vi "获取操作日志 (子VI).vi"(11 "table输入":string(combo)) -> ()   [LabVIEW 2016, in "数据传输系统.lvlib"]
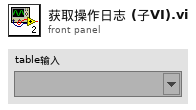
[diagram p1: front panel]
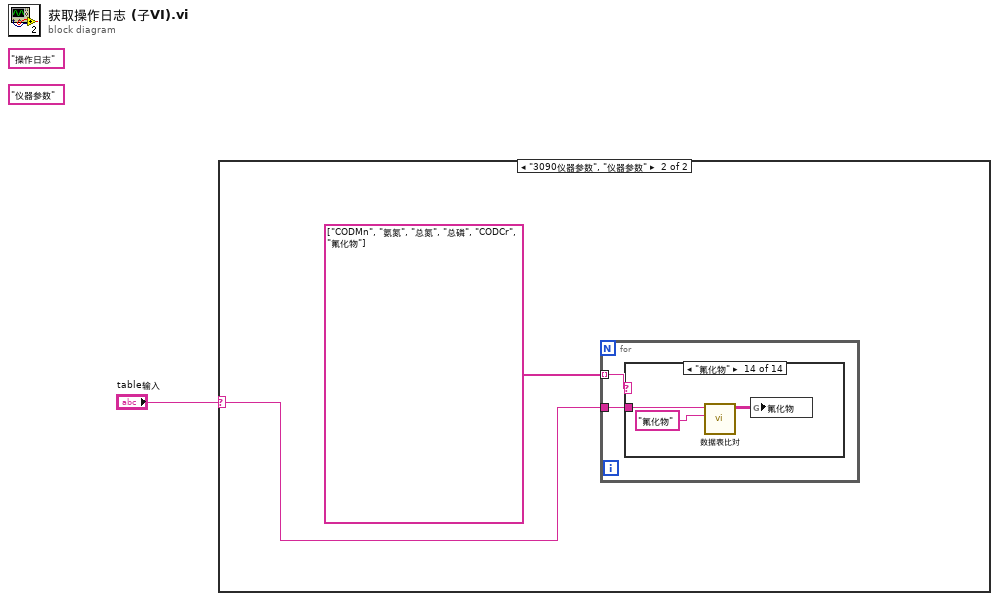
[diagram p0: block diagram]
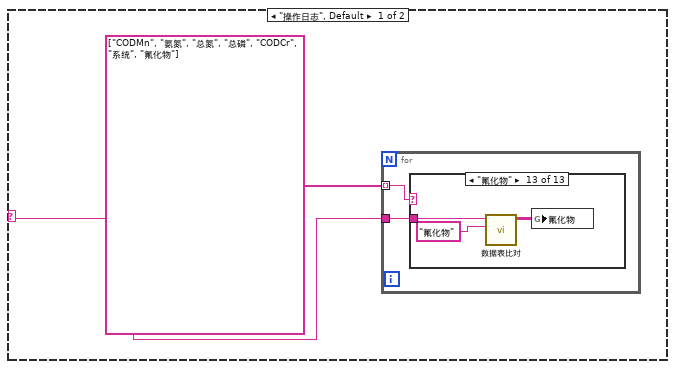
[diagram p2: hidden frame]
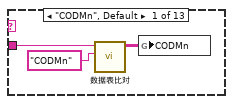
[diagram p3: hidden frame]
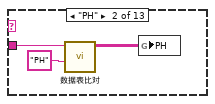
[diagram p4: hidden frame]
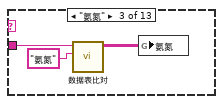
[diagram p5: hidden frame]
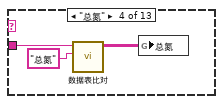
[diagram p6: hidden frame]
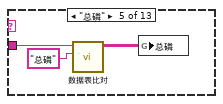
[diagram p7: hidden frame]
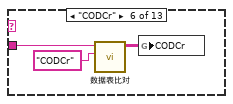
[diagram p8: hidden frame]
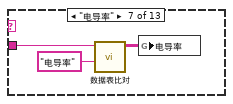
[diagram p9: hidden frame]
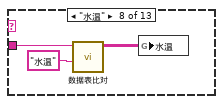
[diagram p10: hidden frame]
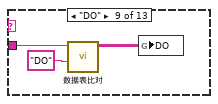
[diagram p11: hidden frame]
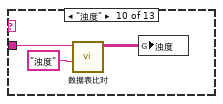
[diagram p12: hidden frame]
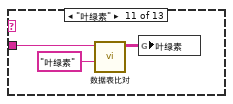
[diagram p13: hidden frame]
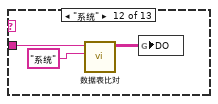
[diagram p14: hidden frame]
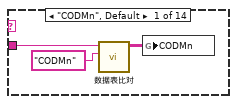
[diagram p15: hidden frame]
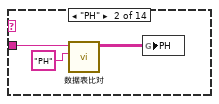
[diagram p16: hidden frame]
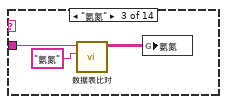
[diagram p17: hidden frame]
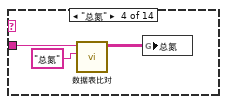
[diagram p18: hidden frame]
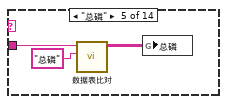
[diagram p19: hidden frame]
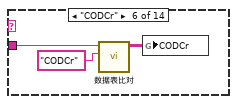
[diagram p20: hidden frame]
diagram:
  (unwired) "仪器参数" ("新元素/子数组")
  (unwired) "操作日志" ("新元素/子数组")
  n1 = case shown="\"3090仪器参数\", \"仪器参数\"" "table输入" {
    selector: "table输入" -> [w2 w45]
    frame "操作日志", Default {
      n2 = for {
        tunnel: string[] ["CODMn", "氨氮", "总氮", "总磷", "CODCr", "系统", "氟化物"] -> [w5] mode=indexing
        tunnel: w2 -> [w4]
        n3 = case shown="\"氟化物\"" w5 {
          tunnel: w4 -> [w6 w9 w12 w15 w18 w21 w24 w27 w30 w33 w36 w39 w42]
          frame "CODMn", Default {
            n4 = call "数据表比对.vi"("仪器日志参数"="CODMn" ("元素"), "table输入"=w6) -> ("待发送数据"=w8:string[][])  [unwired: 6 in, 3 out]
            n5 = global write "全局 所有参数.vi" "CODMn"(w8) -> ()
          }
          frame "PH" {
            n6 = call "数据表比对.vi"("查询元素输入"="PH" ("元素"), "table输入"=w9) -> ("待发送数据"=w10:string[][])  [unwired: 6 in, 3 out]
            n7 = global write "全局 所有参数.vi" "PH"(w10) -> ()
          }
          frame "氨氮" {
            n8 = call "数据表比对.vi"("仪器日志参数"="氨氮" ("元素"), "table输入"=w12) -> ("待发送数据"=w14:string[][])  [unwired: 6 in, 3 out]
            n9 = global write "全局 所有参数.vi" "氨氮"(w14) -> ()
          }
          frame "总氮" {
            n10 = call "数据表比对.vi"("仪器日志参数"="总氮" ("元素"), "table输入"=w15) -> ("待发送数据"=w17:string[][])  [unwired: 6 in, 3 out]
            n11 = global write "全局 所有参数.vi" "总氮"(w17) -> ()
          }
          frame "总磷" {
            n12 = call "数据表比对.vi"("仪器日志参数"="总磷" ("元素"), "table输入"=w18) -> ("待发送数据"=w20:string[][])  [unwired: 6 in, 3 out]
            n13 = global write "全局 所有参数.vi" "总磷"(w20) -> ()
          }
          frame "CODCr" {
            n14 = call "数据表比对.vi"("仪器日志参数"="CODCr" ("元素"), "table输入"=w21) -> ("待发送数据"=w23:string[][])  [unwired: 6 in, 3 out]
            n15 = global write "全局 所有参数.vi" "CODCr"(w23) -> ()
          }
          frame "电导率" {
            n16 = call "数据表比对.vi"("查询元素输入"="电导率" ("元素"), "table输入"=w24) -> ("待发送数据"=w25:string[][])  [unwired: 6 in, 3 out]
            n17 = global write "全局 所有参数.vi" "电导率"(w25) -> ()
          }
          frame "水温" {
            n18 = call "数据表比对.vi"("查询元素输入"="水温" ("元素"), "table输入"=w27) -> ("待发送数据"=w28:string[][])  [unwired: 6 in, 3 out]
            n19 = global write "全局 所有参数.vi" "水温"(w28) -> ()
          }
          frame "DO" {
            n20 = call "数据表比对.vi"("查询元素输入"="DO" ("元素"), "table输入"=w30) -> ("待发送数据"=w31:string[][])  [unwired: 6 in, 3 out]
            n21 = global write "全局 所有参数.vi" "DO"(w31) -> ()
          }
          frame "浊度" {
            n22 = call "数据表比对.vi"("查询元素输入"="浊度" ("元素"), "table输入"=w33) -> ("待发送数据"=w34:string[][])  [unwired: 6 in, 3 out]
            n23 = global write "全局 所有参数.vi" "浊度"(w34) -> ()
          }
          frame "叶绿素" {
            n24 = call "数据表比对.vi"("查询元素输入"="叶绿素" ("元素"), "table输入"=w36) -> ("待发送数据"=w37:string[][])  [unwired: 6 in, 3 out]
            n25 = global write "全局 所有参数.vi" "叶绿素"(w37) -> ()
          }
          frame "系统" {
            n26 = call "数据表比对.vi"("仪器日志参数"="系统" ("元素"), "table输入"=w39) -> ("待发送数据"=w41:string[][])  [unwired: 6 in, 3 out]
            n27 = global write "全局 所有参数.vi" "DO"(w41) -> ()
          }
          frame "氟化物" {
            n28 = call "数据表比对.vi"("仪器日志参数"="氟化物" ("元素"), "table输入"=w42) -> ("待发送数据"=w44:string[][])  [unwired: 6 in, 3 out]
            n29 = global write "全局 所有参数.vi" "氟化物"(w44) -> ()
          }
        }
      }
    }
    frame "3090仪器参数", "仪器参数" {
      n30 = for {
        tunnel: string[] ["CODMn", "氨氮", "总氮", "总磷", "CODCr", "氟化物"] -> [w48] mode=indexing
        tunnel: w45 -> [w47]
        n31 = case shown="\"氟化物\"" w48 {
          tunnel: w47 -> [w49 w53 w55 w58 w61 w64 w68 w71 w74 w77 w80 w82 w85 w88]
          frame "CODMn", Default {
            n32 = call "数据表比对.vi"("仪器日志参数"="CODMn" ("元素"), "table输入"=w49) -> ("待发送数据"=w51:string[][])  [unwired: 6 in, 3 out]
            n33 = global write "全局 所有参数.vi" "CODMn"(w51) -> ()
          }
          frame "PH" {
            n34 = call "数据表比对.vi"("仪器日志参数"="PH" ("元素"), "table输入"=w53) -> ("待发送数据"=w54:string[][])  [unwired: 6 in, 3 out]
            n35 = global write "全局 所有参数.vi" "PH"(w54) -> ()
          }
          frame "氨氮" {
            n36 = call "数据表比对.vi"("仪器日志参数"="氨氮" ("元素"), "table输入"=w55) -> ("待发送数据"=w57:string[][])  [unwired: 6 in, 3 out]
            n37 = global write "全局 所有参数.vi" "氨氮"(w57) -> ()
          }
          frame "总氮" {
            n38 = call "数据表比对.vi"("仪器日志参数"="总氮" ("元素"), "table输入"=w58) -> ("待发送数据"=w60:string[][])  [unwired: 6 in, 3 out]
            n39 = global write "全局 所有参数.vi" "总氮"(w60) -> ()
          }
          frame "总磷" {
            n40 = call "数据表比对.vi"("仪器日志参数"="总磷" ("元素"), "table输入"=w61) -> ("待发送数据"=w63:string[][])  [unwired: 6 in, 3 out]
            n41 = global write "全局 所有参数.vi" "总磷"(w63) -> ()
          }
          frame "CODCr" {
            n42 = call "数据表比对.vi"("仪器日志参数"="CODCr" ("元素"), "table输入"=w64) -> ("待发送数据"=w66:string[][])  [unwired: 6 in, 3 out]
            n43 = global write "全局 所有参数.vi" "CODCr"(w66) -> ()
          }
          frame "电导率" {
            n44 = call "数据表比对.vi"("仪器日志参数"="电导率" ("元素"), "table输入"=w68) -> ("待发送数据"=w69:string[][])  [unwired: 6 in, 3 out]
            n45 = global write "全局 所有参数.vi" "电导率"(w69) -> ()
          }
          frame "水温" {
            n46 = call "数据表比对.vi"("仪器日志参数"="水温" ("元素"), "table输入"=w71) -> ("待发送数据"=w72:string[][])  [unwired: 6 in, 3 out]
            n47 = global write "全局 所有参数.vi" "水温"(w72) -> ()
          }
          frame "DO" {
            n48 = call "数据表比对.vi"("仪器日志参数"="溶解氧" ("元素"), "table输入"=w74) -> ("待发送数据"=w75:string[][])  [unwired: 6 in, 3 out]
            n49 = global write "全局 所有参数.vi" "DO"(w75) -> ()
          }
          frame "浊度" {
            n50 = call "数据表比对.vi"("仪器日志参数"="浊度" ("元素"), "table输入"=w77) -> ("待发送数据"=w78:string[][])  [unwired: 6 in, 3 out]
            n51 = global write "全局 所有参数.vi" "浊度"(w78) -> ()
          }
          frame "叶绿素" {
            n52 = call "数据表比对.vi"("仪器日志参数"="叶绿素" ("元素"), "table输入"=w80) -> ("待发送数据"=w81:string[][])  [unwired: 6 in, 3 out]
            n53 = global write "全局 所有参数.vi" "叶绿素"(w81) -> ()
          }
          frame "藻密度" {
            n54 = call "数据表比对.vi"("仪器日志参数"="藻密度" ("元素"), "table输入"=w82) -> ("待发送数据"=w84:string[][])  [unwired: 6 in, 3 out]
            n55 = global write "全局 所有参数.vi" "藻密度"(w84) -> ()
          }
          frame "ORP" {
            n56 = call "数据表比对.vi"("仪器日志参数"="ORP" ("元素"), "table输入"=w85) -> ("待发送数据"=w87:string[][])  [unwired: 6 in, 3 out]
            n57 = global write "全局 所有参数.vi" "ORP"(w87) -> ()
          }
          frame "氟化物" {
            n58 = call "数据表比对.vi"("仪器日志参数"="氟化物" ("元素"), "table输入"=w88) -> ("待发送数据"=w90:string[][])  [unwired: 6 in, 3 out]
            n59 = global write "全局 所有参数.vi" "氟化物"(w90) -> ()
          }
        }
      }
    }
  }
